vi "Mouse Monitor.vi"(10 "Mouse Up (Outside Pane)":refnum<user-event>, 11 "Initial State":bool[](array[boolean])) -> ()   [LabVIEW 2019]
uses:
  <vilib>/Utility/inputDevices.llb/mouseAcquire.vi
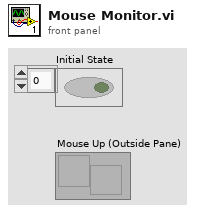
[diagram p1: front panel]
types:
  T1 = cluster{"button 1":bool, "button 2":bool, "button 3":bool, "button 4":bool}
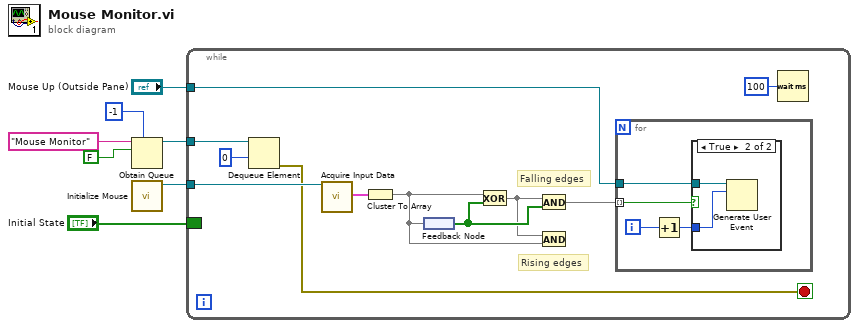
[diagram p0: block diagram]
diagram:
  n1 = Obtain Queue(max queue size (-1, unlimited)=-1, name (unnamed)="Mouse Monitor", element data type=FALSE ("create if not found? (T)")) -> (queue out=w4:refnum<queue>)  [unwired: 2 in, 2 out]
  n2 = call <vilib>:"Initialize Mouse.vi"() -> ("device ID"=w7:refnum<k1>)  [unwired: 10 in, 1 out]
  n3 = while {
    tunnel: w7 -> [w18]
    tunnel: w4 -> [w12]
    border: "Initial State" -> [_]
    tunnel: "Mouse Up (Outside Pane)" -> [w8]
    stop <- w9 stop-if-true
    # "Rising edges"
    # "Falling edges"
    n4 = Dequeue Element(queue=w12, timeout in ms (-1)=0) -> (error out=w9:errorcluster)  [unwired: 1 in, 3 out]
    n5 = call-poly <vilib>:"Acquire Input Data.vi"("device ID"=w18) -> ("button info"=w17:T1)  [unwired: 15 in, 3 out]
    n6 = Cluster To Array(cluster=w17) -> (array=w10:bool[])
    n7 = feedback #1() -> (w16:bool[])
    n8 = feedback-in #1(w10) -> ()
    n9 = Exclusive Or(1:w16, 2:w10) -> (0:w15:bool[])
    n10 = And(x=w15, y=w16) -> (x .and. y?=w14:bool[])
    n11 = And(x=w15, y=w10) -> ()  [unwired: 1 out]
    n12 = for {
      tunnel: w14 -> [w22] mode=indexing
      tunnel: w8 -> [w21]
      i -> [w20]
      n13 = Increment(x=w20) -> (x+1=w19:i32)
      n14 = case shown="True" w22 {
        tunnel: w21 -> [_ w24]
        tunnel: w19 -> [_ w23]
        frame False {
        }
        frame True {
          n15 = Generate User Event(user event=w24, event data cluster=w23) -> ()  [unwired: 2 in, 2 out]
        }
      }
    }
    n16 = Wait (ms)(milliseconds to wait=u32 100) -> ()  [unwired: 1 out]
  }
